vi "Konzentration der einzelnen Komponente umrechnen.vi"(9 "Teilkonzentration":dbl, 10 "Gesamtkonzentration":dbl, 11 "Werteingang":string) -> (3 "Wertausgang":string)   [LabVIEW 2020, in "Linearisierung v2.lvlib" / "Gasteiler.lvlib"]
uses:
  Gasteiler.lvlib
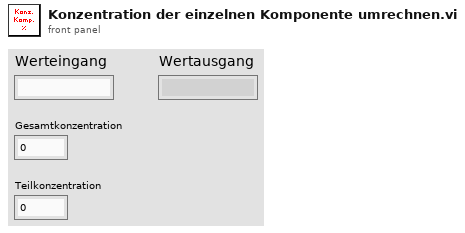
[diagram p1: front panel]
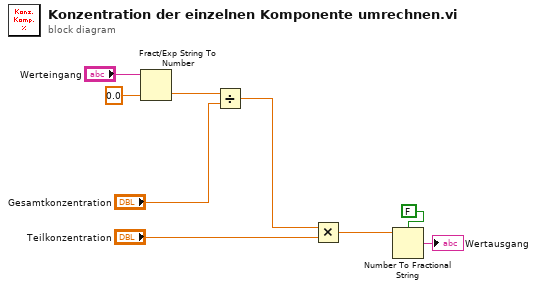
[diagram p0: block diagram]
diagram:
  n1 = Fract/Exp String To Number(string="Werteingang", default (0 dbl)=0.0 ("x")) -> (number=w2:dbl)  [unwired: 2 in, 1 out]
  n2 = Divide(x=w2, y="Gesamtkonzentration") -> (x/y=w1:dbl)
  n3 = Multiply(x=w1, y="Teilkonzentration") -> (x*y=w5:dbl)
  n4 = Number To Fractional String(use system decimal point (T)=FALSE ("Systemdezimalzeichen verwenden (T)"), number=w5) -> (F-format string=→"Wertausgang":string)  [unwired: 2 in]
